vi "Automatic Teller Machine .vi"() -> ()   [LabVIEW 2013]
doc: "This VI is a simulation of Automated Teller Machine controller. The user can interact with control and indicators on the front panel to perform common ATM function like:\n-Inquiry \n-Withdraw\n-Deposit.\n\nAll the user account information is stored in the Account.txt file.\n\nInput can be obtained through:\n-User Input \n-Left and Right Button\n\n-Left and Right Menu manage appropriate action can be taken by pressing left and right button.\n-ATM message indicator will display the message according to the inout pressed\n\nSequence of operation:\n-Start: It runs the application.\n-Isert ATM : Click card simulator,enter account no and verification of account.\n-Deposit: Allow the user to deposit the money.\n-Withdraw: Allow the user to withdraw the money.\n-Fast Cash: User can withdraw 50$.\n-None: Do not produce any result\n-Balance Enquiry: Show the balance remain in the account.\n-Return Card and terminate : It is use for session termination."
uses:
  Controls/ATM States.ctl
  Controls/Function states.ctl
  Controls/Read Write States.ctl
panel:
  in  "Enter":bool
  in  "User Input":string
  in  "Right Buttons":T1
  out "Right Menu":T2
  in  "Left Buttons":T1
  out "Left Menu":T2
  in  "Card Simulator":bool
  out "ATM Messages":string
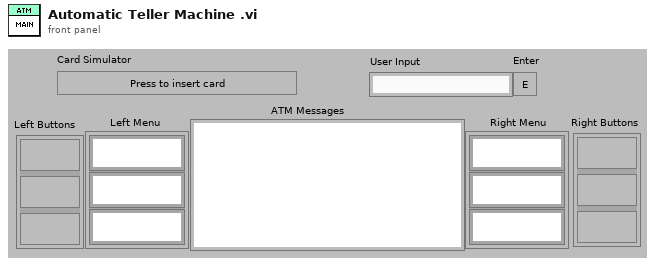
[diagram p1: front panel]
types:
  T1 = cluster{"Func Button":bool, "Func Button 2":bool, "Func Button 3":bool}
  T2 = cluster{"RFS String":string, "RFS String 2":string, "RFS String 3":string}
  T3 = typedef "ATM States.ctl" = enum16{"Initialize", "Card Simulator", "Insert ATM", "Verified", "Ver. failed", "Deposit", "Deposit complete", "Withdraw", "Withdraw complete", "Fast Cash", "Balance Inquiry", "Session Terminate"}
  T4 = typedef "Function states.ctl" = enum16{"Set function", "Get function"}
  T5 = typedef "Read Write States.ctl" = enum16{"Initialize", "Read Data ", "Write Data", "Stop"}
  T6 = enum8{"Enabled", "Disabled", "Disabled and Grayed Out"}
  T7 = cluster{"Name":string, "Company":string, "Acc no.":string, "Balance":i32}
  T8 = cluster{"Name":string, "last Name":string, "Acc no.":string, "Balance":i32}[]
  T9 = cluster{"Name":string, "last Name":string, "Acc no.":string, "Balance":i32}
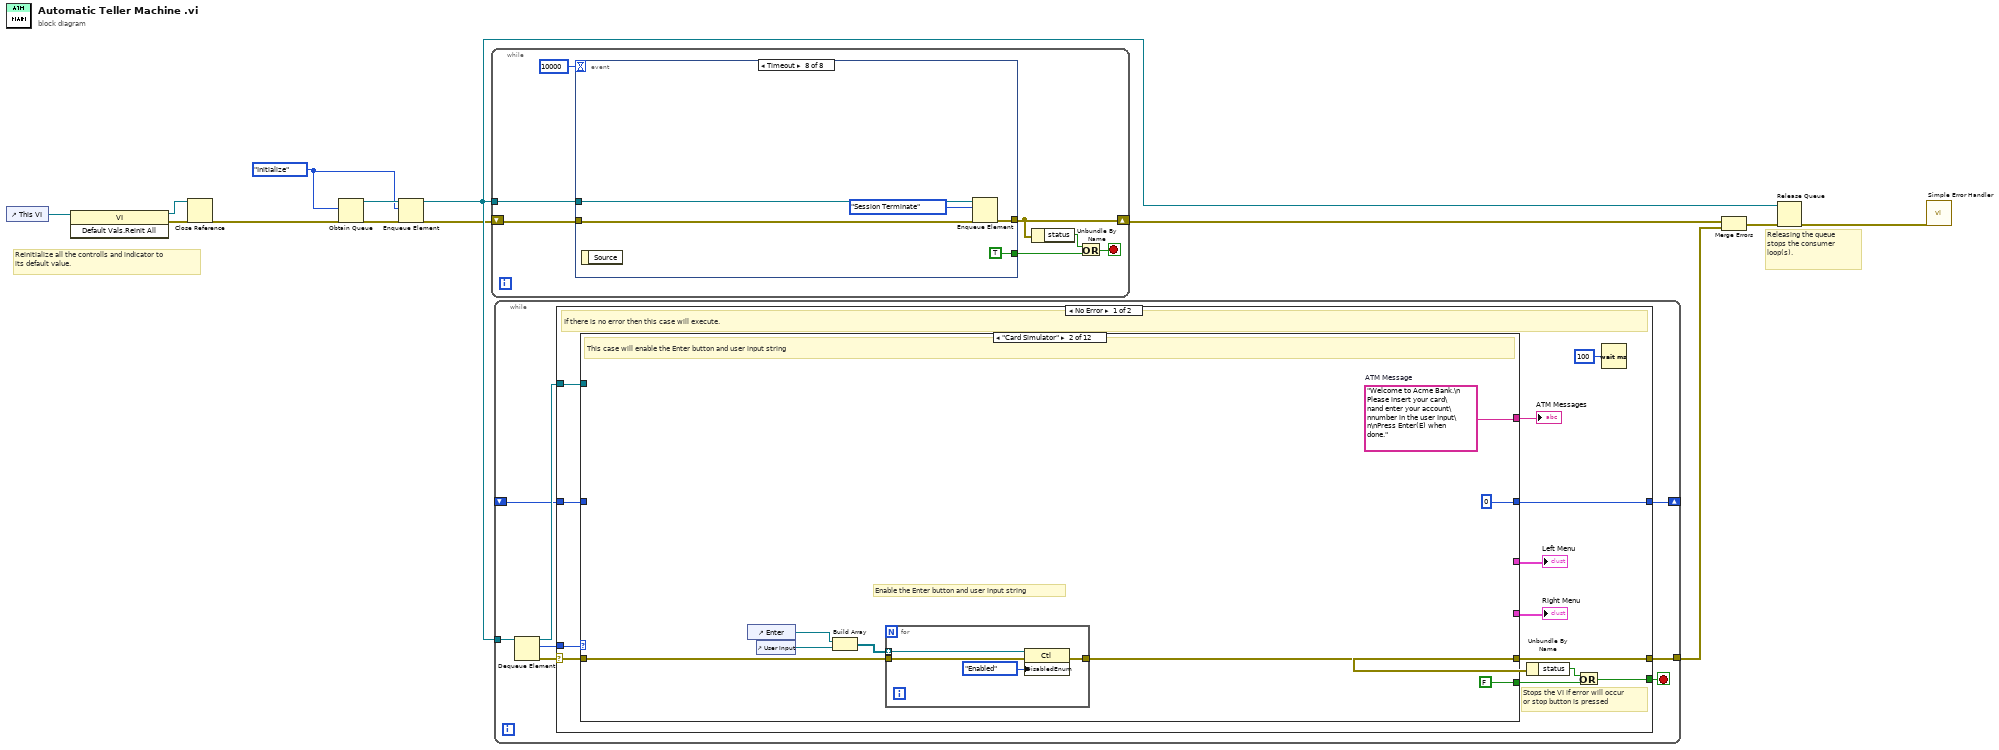
[diagram p0: block diagram]
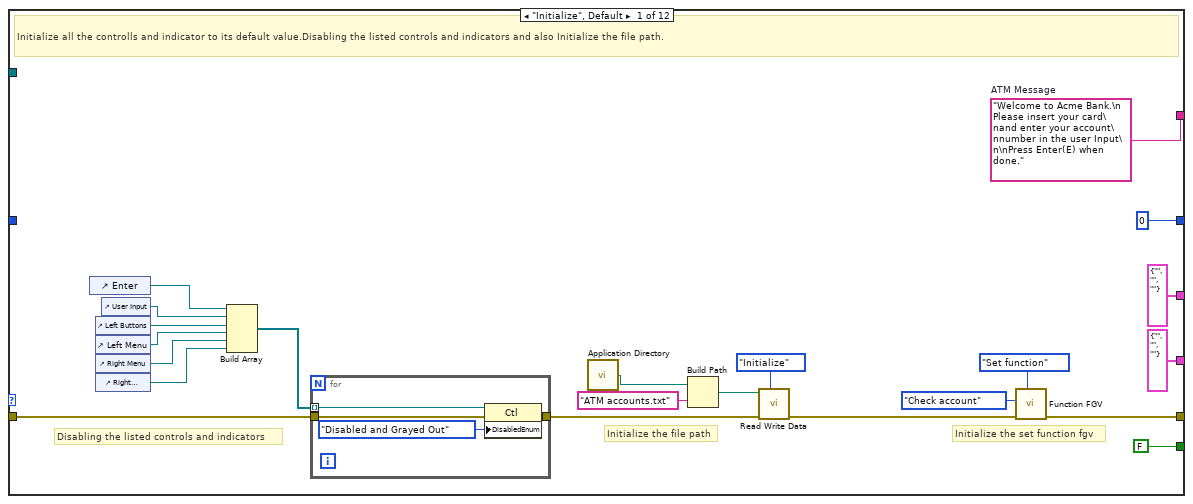
[diagram p2: hidden frame]
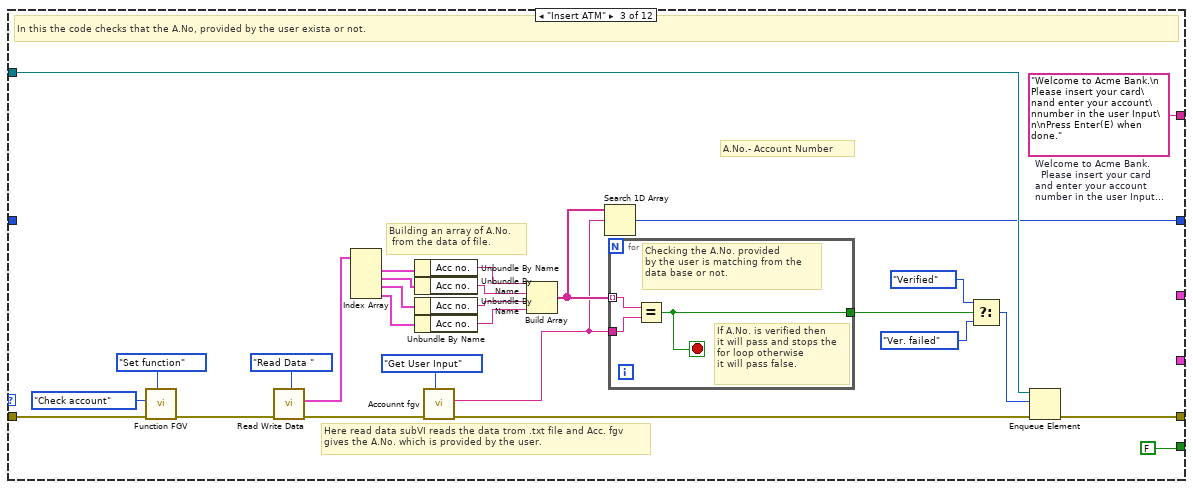
[diagram p3: hidden frame]
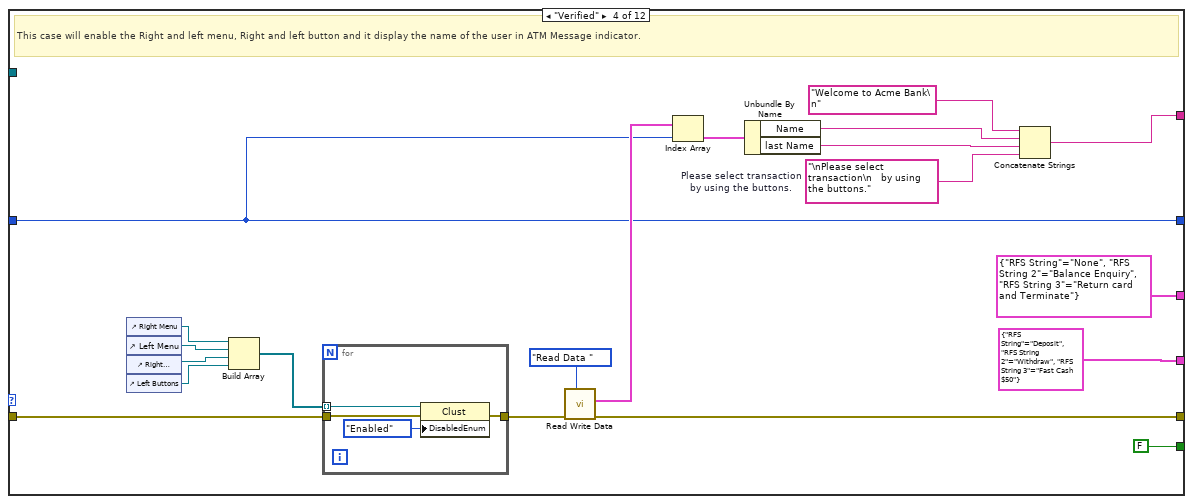
[diagram p4: hidden frame]
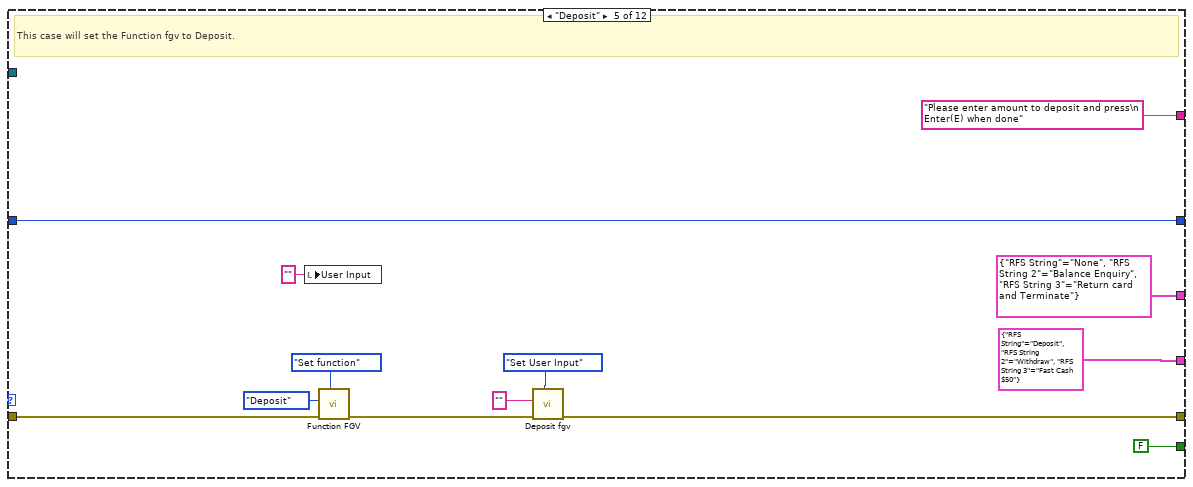
[diagram p5: hidden frame]
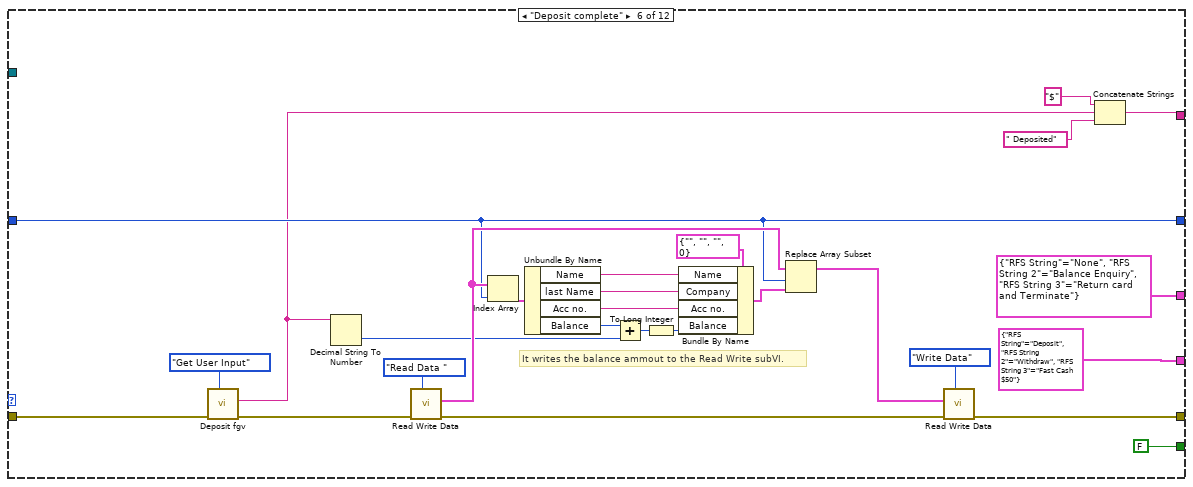
[diagram p6: hidden frame]
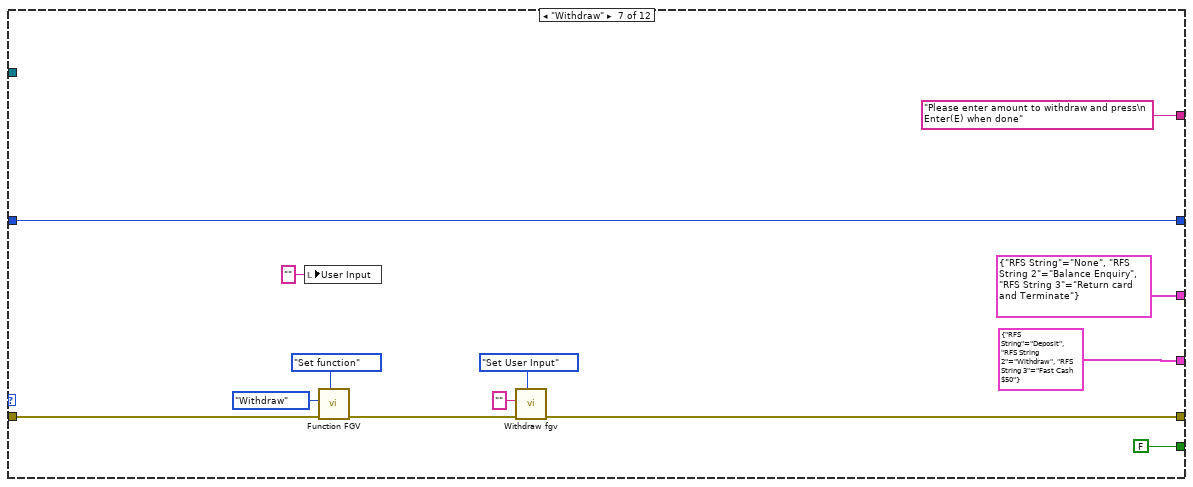
[diagram p7: hidden frame]
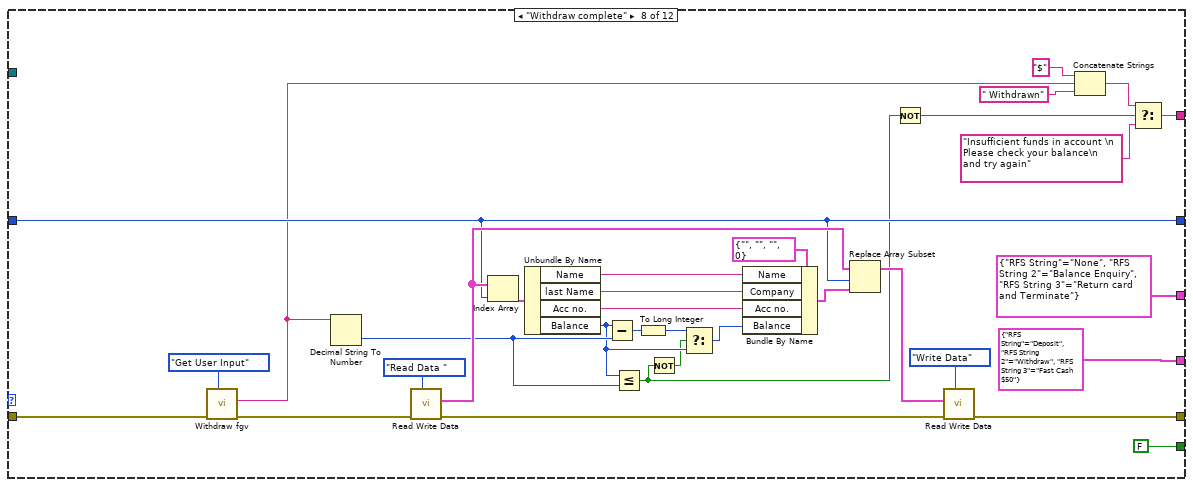
[diagram p8: hidden frame]
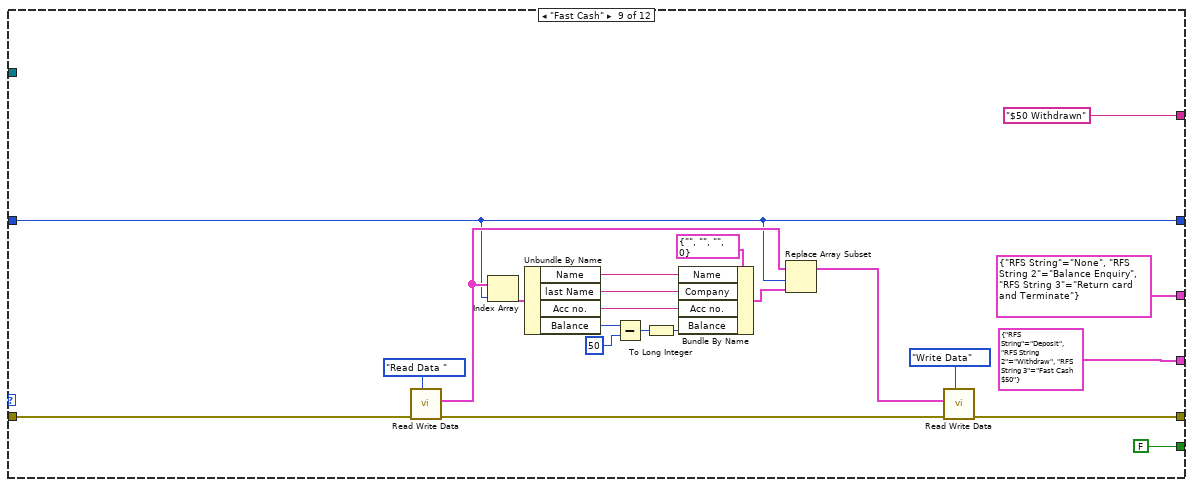
[diagram p9: hidden frame]
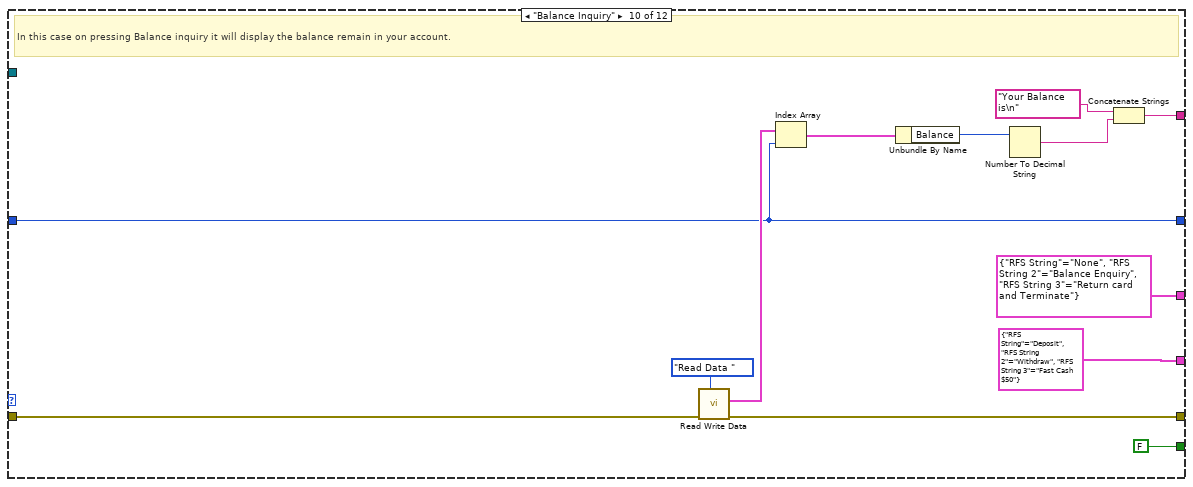
[diagram p10: hidden frame]
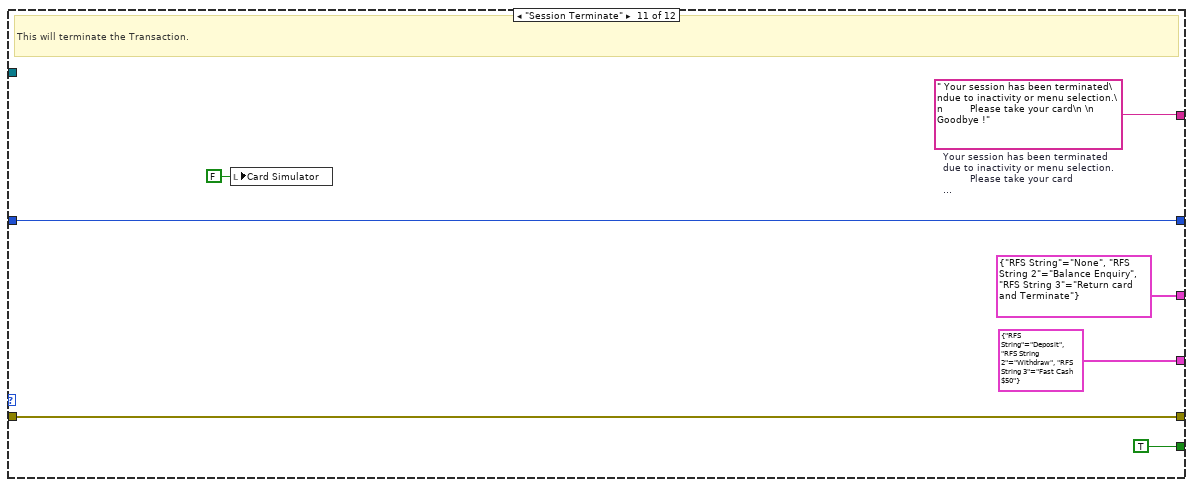
[diagram p11: hidden frame]
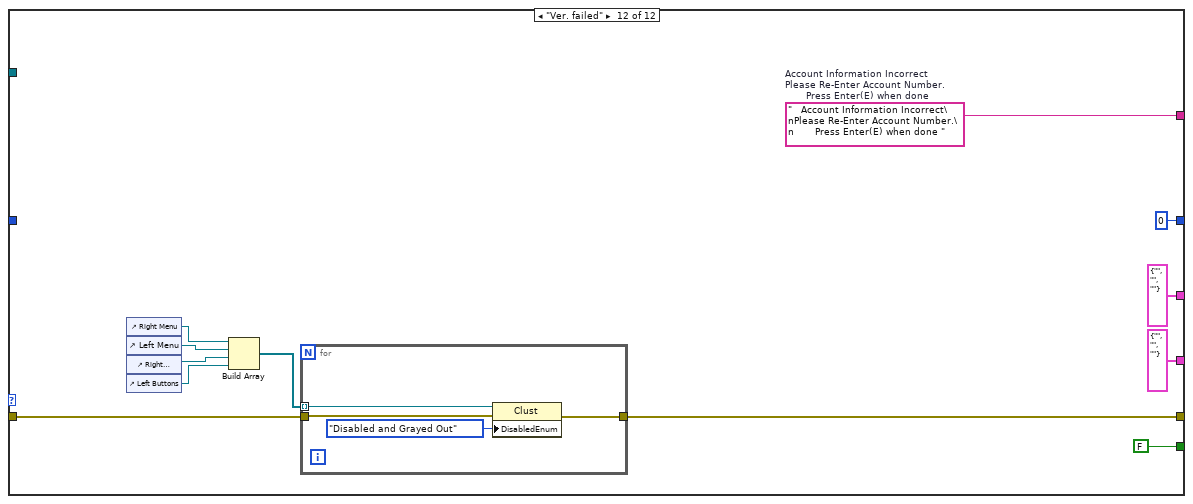
[diagram p12: hidden frame]
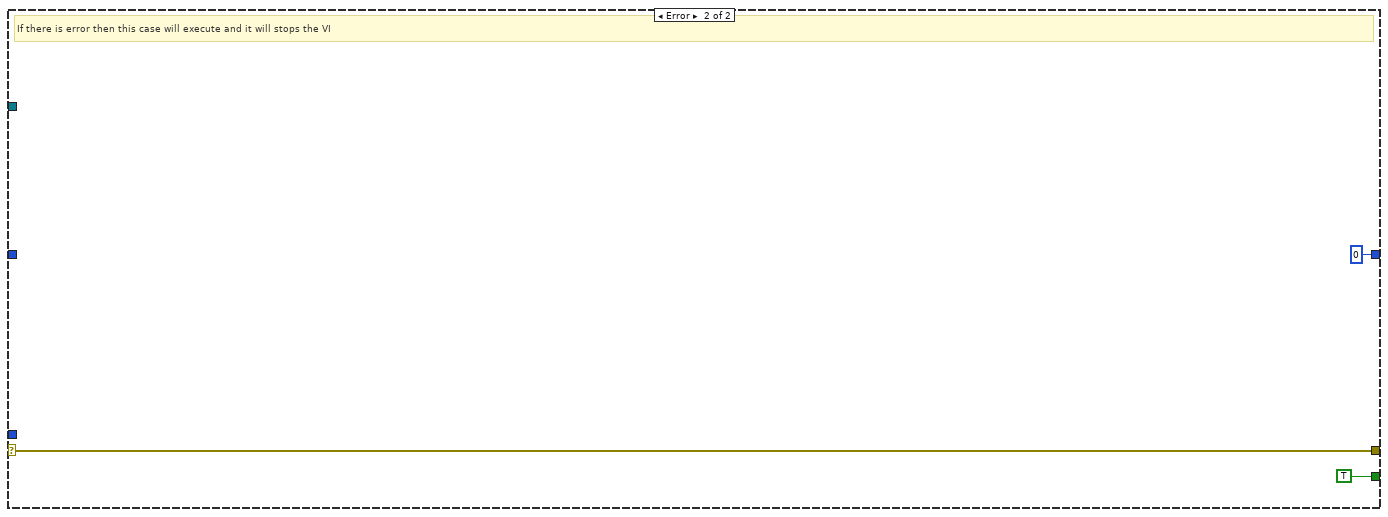
[diagram p13: hidden frame]
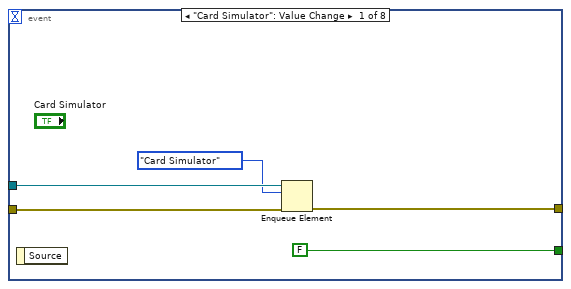
[diagram p14: hidden frame]
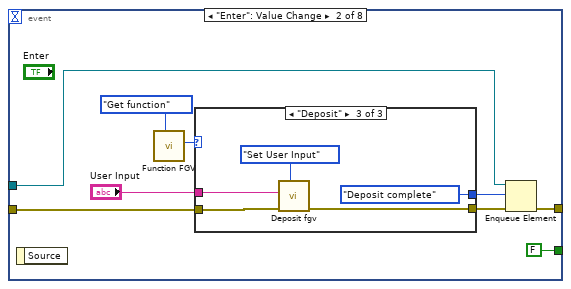
[diagram p15: hidden frame]
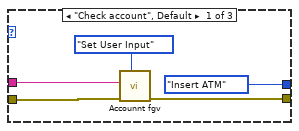
[diagram p16: hidden frame]
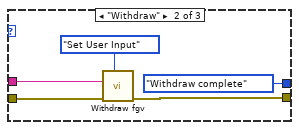
[diagram p17: hidden frame]
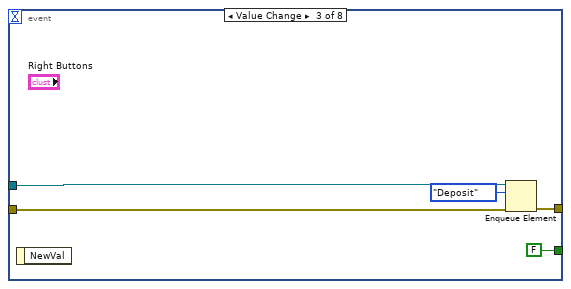
[diagram p18: hidden frame]
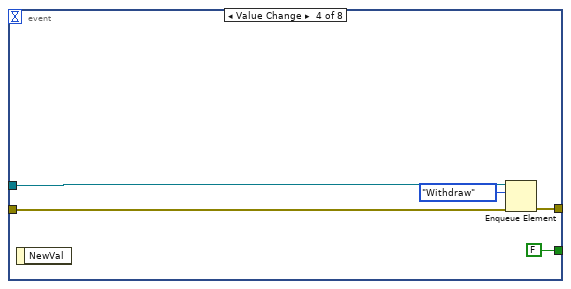
[diagram p19: hidden frame]
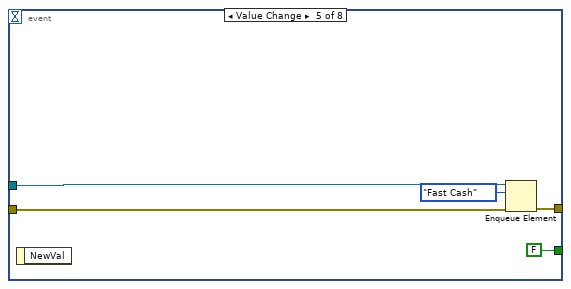
[diagram p20: hidden frame]
diagram:
  w1 = ATM_States."Initialize"
  # "Reinitialize all the controlls and indicator to \nits default value."
  # "Releasing the queue stops the consumer loop(s)."
  n1 = control-ref of="This VI"() -> (w12:refnum<vi>)
  n2 = invoke class="VI" method="Default Vals.Reinit All"(reference=w12) -> (reference out=w10:refnum<vi>, error out=w11:errorcluster)  [unwired: 2 in, 1 out]
  n3 = Close Reference(reference=w10, error in (no error)=w11) -> (error out=w6:errorcluster)
  n4 = Obtain Queue(element data type=w1, error in (no error)=w6) -> (queue out=w13:refnum<queue>, error out=w8:errorcluster)  [unwired: 3 in, 1 out]
  n5 = Enqueue Element(queue=w13, element=w1, error in (no error)=w8) -> (queue out=w9:refnum<queue>, error out=w7:errorcluster)  [unwired: 1 in, 1 out]
  n6 = while {
    shift-right: [w16] -> w2
    shift-left: w7 -> [w19]
    tunnel: w9 -> [w20]
    stop <- w17 stop-if-true
    n7 = event shown="[7] Timeout" {
      selector: _ -> [_ _ _ _ _ _ _ _]
      dyn-events: _ -> [_ _ _ _ _ _ _ _]
      timeout: 10000 -> [_ _ _ _ _ _ _ _]
      tunnel: w20 -> [w25 w27 w51 w56 w61 w66 w71 w76]
      tunnel: w19 -> [w24 w33 w53 w58 w63 w68 w73 w78]
      tunnel: [w23 w28 w52 w57 w62 w67 w72 w77] -> w16
      tunnel: [FALSE FALSE FALSE FALSE FALSE FALSE TRUE TRUE] -> w18
      event "Card Simulator": Value Change {
        n8 = event-data() -> ()  [unwired: 1 in, 1 out]
        n9 = Enqueue Element(queue=w25, element=ATM_States."Card Simulator", error in (no error)=w24) -> (error out=w23:errorcluster)  [unwired: 1 in, 2 out]
      }
      event "Enter": Value Change {
        n10 = event-data() -> ()  [unwired: 1 in, 1 out]
        n11 = call "Function FGV.vi"("Enum 3"=Function_states."Get function") -> ("Enum out"=w32:enum16{"Check account", "Withdraw", "Deposit"})  [unwired: 9 in, 1 out]
        n12 = case shown="\"Deposit\"" w32 {
          tunnel: w33 -> [w39 w44 w49]
          tunnel: [w38 w43 w48] -> w29
          tunnel: "User Input" -> [w36 w42 w46]
          tunnel: [ATM_States."Insert ATM" ("element") ATM_States."Withdraw complete" ("element") ATM_States."Deposit complete" ("element")] -> w26
          frame "Check account", Default {
            n13 = call "Accounnt fgv.vi"("Command"=enum16{"Set User Input", "Get User Input"}."Set User Input", "error in (no error)"=w39, "User Input IN"=w36) -> ("error out"=w38:errorcluster)  [unwired: 7 in, 1 out]
          }
          frame "Withdraw" {
            n14 = call "Withdraw fgv.vi"("Command"=enum16{"Set User Input", "Get User Input"}."Set User Input", "error in (no error)"=w44, "User Input IN  in"=w42) -> ("error out"=w43:errorcluster)  [unwired: 7 in, 1 out]
          }
          frame "Deposit" {
            n15 = call "Deposit fgv.vi"("Command"=enum16{"Set User Input", "Get User Input"}."Set User Input", "error in (no error)"=w49, "User Input IN  in"=w46) -> ("error out"=w48:errorcluster)  [unwired: 7 in, 1 out]
          }
        }
        n16 = Enqueue Element(queue=w27, element=w26, error in (no error)=w29) -> (error out=w28:errorcluster)  [unwired: 1 in, 2 out]
      }
      event "Right Buttons.Func Button": Value Change {
        n17 = event-data() -> ()  [unwired: 1 in, 1 out]
        n18 = Enqueue Element(queue=w51, element=ATM_States."Deposit", error in (no error)=w53) -> (error out=w52:errorcluster)  [unwired: 1 in, 2 out]
      }
      event "Right Buttons.Func Button 2": Value Change {
        n19 = event-data() -> ()  [unwired: 1 in, 1 out]
        n20 = Enqueue Element(queue=w56, element=ATM_States."Withdraw", error in (no error)=w58) -> (error out=w57:errorcluster)  [unwired: 1 in, 2 out]
      }
      event "Right Buttons.Func Button 3": Value Change {
        n21 = event-data() -> ()  [unwired: 1 in, 1 out]
        n22 = Enqueue Element(queue=w61, element=ATM_States."Fast Cash", error in (no error)=w63) -> (error out=w62:errorcluster)  [unwired: 1 in, 2 out]
      }
      event "Left Buttons.Func Button 2": Value Change {
        n23 = event-data() -> ()  [unwired: 1 in, 1 out]
        n24 = Enqueue Element(queue=w66, element=ATM_States."Balance Inquiry", error in (no error)=w68) -> (error out=w67:errorcluster)  [unwired: 1 in, 2 out]
      }
      event "Left Buttons.Func Button 3": Value Change {
        n25 = event-data() -> ()  [unwired: 1 in, 1 out]
        n26 = Enqueue Element(queue=w71, element=ATM_States."Session Terminate", error in (no error)=w73) -> (error out=w72:errorcluster)  [unwired: 1 in, 2 out]
      }
      event Timeout {
        n27 = event-data() -> ()  [unwired: 1 in, 1 out]
        n28 = Enqueue Element(queue=w76, element=ATM_States."Session Terminate", error in (no error)=w78) -> (error out=w77:errorcluster)  [unwired: 1 in, 2 out]
      }
    }
    n29 = Unbundle By Name(w16) -> ("status"=w15:bool)
    n30 = Or(x=w15, y=w18) -> (x .or. y?=w17:bool)
  }
  n31 = while {
    tunnel: w9 -> [w87]
    tunnel: [w83] -> w3
    shift-right: [w81] -> _
    shift-left: _ -> [w80]
    stop <- w84 stop-if-true
    n32 = Dequeue Element(queue=w87) -> (queue out=w82:refnum<queue>, element=w85:T3, error out=w86:errorcluster)  [unwired: 2 in, 1 out]
    n33 = case shown="No Error" w86 {
      selector: w86 -> [w100 w339]
      tunnel: w85 -> [w95 _]
      tunnel: [w98 TRUE] -> w84
      tunnel: [w99 w339] -> w83
      tunnel: w82 -> [w93 _]
      tunnel: [w92 0 ("index of element")] -> w81
      tunnel: w80 -> [w91 _]
      frame No Error {
        # "Stops the VI if error will occur\nor stop button is pressed"
        # "If there is no error then this case will execute."
        n34 = case shown="\"Card Simulator\"" w95 {
          tunnel: [w105 w129 w146 w181 w196 w229 w241 w275 w296 w311 w317 w325] -> w99
          tunnel: w100 -> [w114 w130 w165 w183 w198 w211 w235 w260 w281 w306 w317 w326]
          tunnel: [FALSE FALSE FALSE FALSE FALSE FALSE FALSE FALSE FALSE FALSE TRUE FALSE] -> w96
          tunnel: [w122 w134 w149 w176 "Please enter amount to deposit and press\n                    Enter(E) when done" w208 "Please enter amount to withdraw and press\n                    Enter(E) when done" w253 "$50 Withdrawn" w302 w316 w333] -> w94
          tunnel: w93 -> [_ _ w145 _ _ _ _ _ _ _ _ _]
          tunnel: [0 ("index of element") 0 ("index of element") w139 w175 w205 w221 w245 w269 w290 w308 w318 0 ("index of element")] -> w92
          tunnel: w91 -> [_ _ _ w175 w205 w221 w245 w269 w290 w308 w318 _]
          tunnel: [T2 {"RFS String"="", "RFS String 2"="", "RFS String 3"=""} ("Left Menu") _ _ T2 {"RFS String"="None", "RFS String 2"="Balance Enquiry", "RFS String 3"="Return card and Terminate"} ("Left Menu") T2 {"RFS String"="None", "RFS String 2"="Balance Enquiry", "RFS String 3"="Return card and Terminate"} ("Left Menu") T2 {"RFS String"="None", "RFS String 2"="Balance Enquiry", "RFS String 3"="Return card and Terminate"} ("Left Menu") T2 {"RFS String"="None", "RFS String 2"="Balance Enquiry", "RFS String 3"="Return card and Terminate"} ("Left Menu") T2 {"RFS String"="None", "RFS String 2"="Balance Enquiry", "RFS String 3"="Return card and Terminate"} ("Left Menu") T2 {"RFS String"="None", "RFS String 2"="Balance Enquiry", "RFS String 3"="Return card and Terminate"} ("Left Menu") T2 {"RFS String"="None", "RFS String 2"="Balance Enquiry", "RFS String 3"="Return card and Terminate"} ("Left Menu") T2 {"RFS String"="None", "RFS String 2"="Balance Enquiry", "RFS String 3"="Return card and Terminate"} ("Left Menu") T2 {"RFS String"="", "RFS String 2"="", "RFS String 3"=""} ("Left Menu")] -> w90
          tunnel: [T2 {"RFS String"="", "RFS String 2"="", "RFS String 3"=""} ("Right Menu") _ _ T2 {"RFS String"="Deposit", "RFS String 2"="Withdraw", "RFS String 3"="Fast Cash $50"} ("Right Menu") T2 {"RFS String"="Deposit", "RFS String 2"="Withdraw", "RFS String 3"="Fast Cash $50"} ("Right Menu") T2 {"RFS String"="Deposit", "RFS String 2"="Withdraw", "RFS String 3"="Fast Cash $50"} ("Right Menu") T2 {"RFS String"="Deposit", "RFS String 2"="Withdraw", "RFS String 3"="Fast Cash $50"} ("Right Menu") T2 {"RFS String"="Deposit", "RFS String 2"="Withdraw", "RFS String 3"="Fast Cash $50"} ("Right Menu") T2 {"RFS String"="Deposit", "RFS String 2"="Withdraw", "RFS String 3"="Fast Cash $50"} ("Right Menu") T2 {"RFS String"="Deposit", "RFS String 2"="Withdraw", "RFS String 3"="Fast Cash $50"} ("Right Menu") T2 {"RFS String"="Deposit", "RFS String 2"="Withdraw", "RFS String 3"="Fast Cash $50"} ("Right Menu") T2 {"RFS String"="", "RFS String 2"="", "RFS String 3"=""} ("Right Menu")] -> w89
          frame "Initialize", Default {
            w122 = "Welcome to Acme Bank.\n  Please insert your card\nand enter your account\nnumber in the user Input\n\nPress Enter(E) when done."  # ATM Message
            # "Initialize the set function fgv"
            # "Disabling the listed controls and indicators"
            # "Initialize the file path"
            # "Initialize all the controlls and indicator to its default value.Disabling the listed controls and indicators and also Initialize the file path."
            n35 = control-ref of="Enter"() -> (w121:refnum<vi>)
            n36 = control-ref of="Left Buttons"() -> (w119:refnum<vi>)
            n37 = control-ref of="Left Menu"() -> (w118:refnum<vi>)
            n38 = control-ref of="Right Menu"() -> (w117:refnum<vi>)
            n39 = control-ref of="Right Buttons"() -> (w116:refnum<vi>)
            n40 = control-ref of="User Input"() -> (w120:refnum<vi>)
            n41 = Build Array(w121, w120, w119, w118, w117, w116) -> (w115:refnum<vi>[])
            n42 = for {
              tunnel: w115 -> [w126] mode=indexing
              tunnel: w114 -> [w124]
              tunnel: [w123] -> w113
              n43 = property on="Property Node" class="Ctl"(reference=w126, error in=w124, "DisabledEnum"=T6."Disabled and Grayed Out" ("Disabled")) -> (error out=w123:errorcluster)  [unwired: 1 out]
            }
            n44 = call <vilib>:"Application Directory.vi"() -> ("Application Directory"=w111:path)
            n45 = Build Path(base path=w111, name or relative path="ATM accounts.txt") -> (appended path=w109:path)
            n46 = call "Read Write Data.vi"("Command"=Read_Write_States."Initialize", "error in (no error)"=w113, "file path"=w109) -> ("error IO"=w106:errorcluster)  [unwired: 7 in, 1 out]
            n47 = call "Function FGV.vi"("Enum 3"=Function_states."Set function", "error constant"=w106, "Enum in"=enum16{"Check account", "Withdraw", "Deposit"}."Check account") -> ("error IO"=w105:errorcluster)  [unwired: 7 in, 1 out]
          }
          frame "Card Simulator" {
            w134 = "Welcome to Acme Bank.\n  Please insert your card\nand enter your account\nnumber in the user Input\n\nPress Enter(E) when done."  # ATM Message
            # "Enable the Enter button and user input string"
            # "This case will enable the Enter button and user input string"
            n48 = control-ref of="Enter"() -> (w133:refnum<vi>)
            n49 = control-ref of="User Input"() -> (w132:refnum<vi>)
            n50 = Build Array(w133, w132) -> (w131:refnum<vi>[])
            n51 = for {
              tunnel: w131 -> [w138] mode=indexing
              tunnel: w130 -> [w136]
              tunnel: [w135] -> w129
              n52 = property on="Property Node" class="Ctl"(reference=w138, error in=w136, "DisabledEnum"=T6."Enabled" ("Disabled")) -> (error out=w135:errorcluster)  [unwired: 1 out]
            }
          }
          frame "Insert ATM" {
            w149 = "Welcome to Acme Bank.\n  Please insert your card\nand enter your account\nnumber in the user Input\n\nPress Enter(E) when done."  # Welcome to Acme Bank.   Please insert your card and enter your account number in the user Input  Press Enter(E) when done.
            # "A.No.- Account Number"
            # "Building an array of A.No.\n from the data of file."
            # "Here read data subVI reads the data trom .txt file and Acc. fgv \ngives the A.No. which is provided by the user."
            # "In this the code checks that the A.No, provided by the user exista or not."
            n53 = call "Function FGV.vi"("Enum 3"=Function_states."Set function", "error constant"=w165, "Enum in"=enum16{"Check account", "Withdraw", "Deposit"}."Check account") -> ("error IO"=w160:errorcluster)  [unwired: 7 in, 1 out]
            n54 = call "Read Write Data.vi"("Command"=Read_Write_States."Read Data ", "error in (no error)"=w160) -> ("error IO"=w159:errorcluster, "Array out"=w158:T8)  [unwired: 8 in]
            n55 = Index Array(array=w158) -> (element #1=w157:T9, element #2=w156:T9, element #3=w155:T9, element #4=w154:T9)  [unwired: 4 in]
            n56 = Unbundle By Name(w157) -> ("Acc no."=w153:string)
            n57 = Unbundle By Name(w156) -> ("Acc no."=w151:string)
            n58 = Unbundle By Name(w155) -> ("Acc no."=w150:string)
            n59 = Unbundle By Name(w154) -> ("Acc no."=w152:string)
            n60 = call "Accounnt fgv.vi"("Command"=enum16{"Set User Input", "Get User Input"}."Get User Input", "error in (no error)"=w159) -> ("error out"=w147:errorcluster, "User Input OUT"=w140:string)  [unwired: 8 in]
            n61 = Build Array(w153, w151, w150, w152) -> (w141:string[])
            n62 = Search 1D Array(1D array=w141, element=w140) -> (index of element=w139:i32)  [unwired: 1 in]
            n63 = for {
              tunnel: w141 -> [w169] mode=indexing
              tunnel: w140 -> [w168]
              tunnel: [w167] -> w148
              stop <- w167 stop-if-true
              # "If A.No. is verified then\nit will pass and stops the \nfor loop otherwise\nit will pass false."
              # "Checking the A.No. provided \nby the user is matching from the \ndata base or not."
              n64 = Equal?(x=w169, y=w168) -> (x = y?=w167:bool)
            }
            n65 = Select(t=ATM_States."Verified" ("element"), s=w148, f=ATM_States."Ver. failed" ("element")) -> (s? t:f=w142:T3)
            n66 = Enqueue Element(queue=w145, element=w142, error in (no error)=w147) -> (error out=w146:errorcluster)  [unwired: 1 in, 2 out]
          }
          frame "Verified" {
            w174 = "\nPlease select transaction\n   by using the buttons."  # Please select transaction    by using the buttons.
            # "This case will enable the Right and left menu, Right and left button and it display the name of the user in ATM Message indicator."
            n67 = control-ref of="Right Menu"() -> (w188:refnum<vi>)
            n68 = control-ref of="Left Menu"() -> (w187:refnum<vi>)
            n69 = control-ref of="Right Buttons"() -> (w185:refnum<vi>)
            n70 = control-ref of="Left Buttons"() -> (w186:refnum<vi>)
            n71 = Build Array(w188, w187, w185, w186) -> (w184:refnum<vi>[])
            n72 = for {
              tunnel: w184 -> [w193] mode=indexing
              tunnel: w183 -> [w192]
              tunnel: [w191] -> w182
              n73 = property on="Property Node" class="Clust"(reference=w193, error in=w192, "DisabledEnum"=T6."Enabled" ("Disabled")) -> (error out=w191:errorcluster)  [unwired: 1 out]
            }
            n74 = call "Read Write Data.vi"("Command"=Read_Write_States."Read Data ", "error in (no error)"=w182) -> ("error IO"=w181:errorcluster, "Array out"=w179:T8)  [unwired: 8 in]
            n75 = Index Array(array=w179, index=w175) -> (element=w178:T9)
            n76 = Unbundle By Name(w178) -> ("Name"=w172:string, "last Name"=w173:string)
            n77 = Concatenate Strings("Welcome to Acme Bank\n", w172, w173, w174) -> (w176:string)
          }
          frame "Deposit" {
            # "This case will set the Function fgv to Deposit."
            n78 = local write "User Input"("" ("User Input")) -> ()
            n79 = call "Function FGV.vi"("Enum 3"=Function_states."Set function", "error constant"=w198, "Enum in"=enum16{"Check account", "Withdraw", "Deposit"}."Deposit") -> ("error IO"=w197:errorcluster)  [unwired: 7 in, 1 out]
            n80 = call "Deposit fgv.vi"("Command"=enum16{"Set User Input", "Get User Input"}."Set User Input", "error in (no error)"=w197, "User Input IN  in"="") -> ("error out"=w196:errorcluster)  [unwired: 7 in, 1 out]
          }
          frame "Deposit complete" {
            # "It writes the balance ammout to the Read Write subVI."
            n81 = call "Deposit fgv.vi"("Command"=enum16{"Set User Input", "Get User Input"}."Get User Input", "error in (no error)"=w211) -> ("error out"=w227:errorcluster, "User Input IN  out"=w209:string)  [unwired: 8 in]
            n82 = Decimal String To Number(string=w209) -> (number=w216:i32)  [unwired: 2 in, 1 out]
            n83 = call "Read Write Data.vi"("Command"=Read_Write_States."Read Data ", "error in (no error)"=w227) -> ("error IO"=w226:errorcluster, "Array out"=w222:T8)  [unwired: 8 in]
            n84 = Index Array(array=w222, index=w221) -> (element=w220:T9)
            n85 = Unbundle By Name(w220) -> ("Name"=w214:string, "last Name"=w213:string, "Acc no."=w212:string, "Balance"=w217:i32)
            n86 = Add(x=w217, y=w216) -> (x+y=w219:i32)
            n87 = To Long Integer(number=w219) -> (32bit integer=w218:i32)
            n88 = Bundle By Name(cluster=T7 {"Name"="", "Company"="", "Acc no."="", "Balance"=0} ("data In  2"), "Name"=w214, "Company"=w213, "Acc no."=w212, "Balance"=w218) -> (w224:T7)
            n89 = Replace Array Subset(array=w222, new element=w224, index=w221) -> (w215:T8)
            n90 = call "Read Write Data.vi"("Command"=Read_Write_States."Write Data", "error in (no error)"=w226, "Array In"=w215) -> ("error IO"=w229:errorcluster)  [unwired: 7 in, 1 out]
            n91 = Concatenate Strings("$" ("string"), w209, " Deposited") -> (w208:string)
          }
          frame "Withdraw" {
            n92 = local write "User Input"("" ("User Input")) -> ()
            n93 = call "Function FGV.vi"("Enum 3"=Function_states."Set function", "error constant"=w235, "Enum in"=enum16{"Check account", "Withdraw", "Deposit"}."Withdraw") -> ("error IO"=w234:errorcluster)  [unwired: 7 in, 1 out]
            n94 = call "Withdraw fgv.vi"("Command"=enum16{"Set User Input", "Get User Input"}."Set User Input", "error in (no error)"=w234, "User Input IN  in"="") -> ("error out"=w241:errorcluster)  [unwired: 7 in, 1 out]
          }
          frame "Withdraw complete" {
            n95 = call "Withdraw fgv.vi"("Command"=enum16{"Set User Input", "Get User Input"}."Get User Input", "error in (no error)"=w260) -> ("error out"=w259:errorcluster, "User Input IN  out"=w258:string)  [unwired: 8 in]
            n96 = Decimal String To Number(string=w258) -> (number=w254:i32)  [unwired: 2 in, 1 out]
            n97 = call "Read Write Data.vi"("Command"=Read_Write_States."Read Data ", "error in (no error)"=w259) -> ("error IO"=w274:errorcluster, "Array out"=w270:T8)  [unwired: 8 in]
            n98 = Index Array(array=w270, index=w269) -> (element=w268:T9)
            n99 = Unbundle By Name(w268) -> ("Name"=w265:string, "last Name"=w264:string, "Acc no."=w263:string, "Balance"=w249:i32)
            n100 = Subtract(x=w249, y=w254) -> (x-y=w267:i32)
            n101 = Less Or Equal?(x=w249, y=w254) -> (x <= y?=w251:bool)
            n102 = To Long Integer(number=w267) -> (32bit integer=w250:i32)
            n103 = Not(x=w251) -> (.not. x?=w247:bool)
            n104 = Select(t=w250, s=w247, f=w249) -> (s? t:f=w248:i32)
            n105 = Bundle By Name(cluster=T7 {"Name"="", "Company"="", "Acc no."="", "Balance"=0} ("data In  2"), "Name"=w265, "Company"=w264, "Acc no."=w263, "Balance"=w248) -> (w272:T7)
            n106 = Replace Array Subset(array=w270, new element=w272, index=w269) -> (w266:T8)
            n107 = Not(x=w251) -> (.not. x?=w252:bool)
            n108 = call "Read Write Data.vi"("Command"=Read_Write_States."Write Data", "error in (no error)"=w274, "Array In"=w266) -> ("error IO"=w275:errorcluster)  [unwired: 7 in, 1 out]
            n109 = Concatenate Strings("$" ("string"), w258, " Withdrawn") -> (w256:string)
            n110 = Select(t=w256, s=w252, f="Insufficient funds in account \n   Please check your balance\n            and try again") -> (s? t:f=w253:string)
          }
          frame "Fast Cash" {
            n111 = call "Read Write Data.vi"("Command"=Read_Write_States."Read Data ", "error in (no error)"=w281) -> ("error IO"=w295:errorcluster, "Array out"=w291:T8)  [unwired: 8 in]
            n112 = Index Array(array=w291, index=w290) -> (element=w289:T9)
            n113 = Unbundle By Name(w289) -> ("Name"=w284:string, "last Name"=w283:string, "Acc no."=w282:string, "Balance"=w286:i32)
            n114 = Subtract(x=w286, y=50) -> (x-y=w288:i32)
            n115 = To Long Integer(number=w288) -> (32bit integer=w287:i32)
            n116 = Bundle By Name(cluster=T7 {"Name"="", "Company"="", "Acc no."="", "Balance"=0} ("data In  2"), "Name"=w284, "Company"=w283, "Acc no."=w282, "Balance"=w287) -> (w293:T7)
            n117 = Replace Array Subset(array=w291, new element=w293, index=w290) -> (w285:T8)
            n118 = call "Read Write Data.vi"("Command"=Read_Write_States."Write Data", "error in (no error)"=w295, "Array In"=w285) -> ("error IO"=w296:errorcluster)  [unwired: 7 in, 1 out]
          }
          frame "Balance Inquiry" {
            # "In this case on pressing Balance inquiry it will display the balance remain in your account."
            n119 = call "Read Write Data.vi"("Command"=Read_Write_States."Read Data ", "error in (no error)"=w306) -> ("error IO"=w311:errorcluster, "Array out"=w309:T8)  [unwired: 8 in]
            n120 = Index Array(array=w309, index=w308) -> (element=w307:T9)
            n121 = Unbundle By Name(w307) -> ("Balance"=w305:i32)
            n122 = Number To Decimal String(number=w305) -> (decimal integer string=w303:string)  [unwired: 1 in]
            n123 = Concatenate Strings("Your Balance is\n", w303) -> (w302:string)
          }
          frame "Session Terminate" {
            w316 = " Your session has been terminated\ndue to inactivity or menu selection.\n         Please take your card\n \n              Goodbye !"  # Your session has been terminated due to inactivity or menu selection.          Please take your card                 Goodbye !
            # "This will terminate the Transaction."
            n124 = local write "Card Simulator"(FALSE ("Card Simulator")) -> ()
          }
          frame "Ver. failed" {
            w333 = "   Account Information Incorrect\nPlease Re-Enter Account Number.\n       Press Enter(E) when done "  # Account Information Incorrect Please Re-Enter Account Number.        Press Enter(E) when done
            n125 = control-ref of="Right Menu"() -> (w331:refnum<vi>)
            n126 = control-ref of="Left Menu"() -> (w330:refnum<vi>)
            n127 = control-ref of="Right Buttons"() -> (w328:refnum<vi>)
            n128 = control-ref of="Left Buttons"() -> (w329:refnum<vi>)
            n129 = Build Array(w331, w330, w328, w329) -> (w327:refnum<vi>[])
            n130 = for {
              tunnel: w327 -> [w337] mode=indexing
              tunnel: w326 -> [w336]
              tunnel: [w335] -> w325
              n131 = property on="Property Node" class="Clust"(reference=w337, error in=w336, "DisabledEnum"=T6."Disabled and Grayed Out" ("Disabled")) -> (error out=w335:errorcluster)  [unwired: 1 out]
            }
          }
        }
        "ATM Messages" <- w94
        "Left Menu" <- w90
        "Right Menu" <- w89
        n132 = Unbundle By Name(w99) -> ("status"=w97:bool)
        n133 = Or(x=w97, y=w96) -> (x .or. y?=w98:bool)
        n134 = Wait (ms)(milliseconds to wait=u32 100) -> ()  [unwired: 1 out]
      }
      frame Error {
        # "If there is error then this case will execute and it will stops the VI"
      }
    }
  }
  n135 = Merge Errors(w2, w3) -> (w5:errorcluster)
  n136 = Release Queue(queue=w9, error in (no error)=w5) -> (error out=w4:errorcluster)  [unwired: 1 in, 2 out]
  n137 = call <vilib>:"Simple Error Handler.vi"("error in (no error)"=w4) -> ()  [unwired: 4 in, 5 out]
